vi "Mu_Variance_linearCombinaison.vi"(11 "elements":cluster{"Intensity Graph 3":u8[][]}[][](array[cluster])) -> ()   [LabVIEW 2018, in "statistics.lvlib"]
uses:
  statistics.lvlib
panel:
  in  "Hologram array":dbl[](array[numeric])=[0.0, 0.25, 0.5, 0.75]
  out "subarray":cluster{"Intensity Graph 3":u8[][]}[](array[cluster])
  out "element":i32
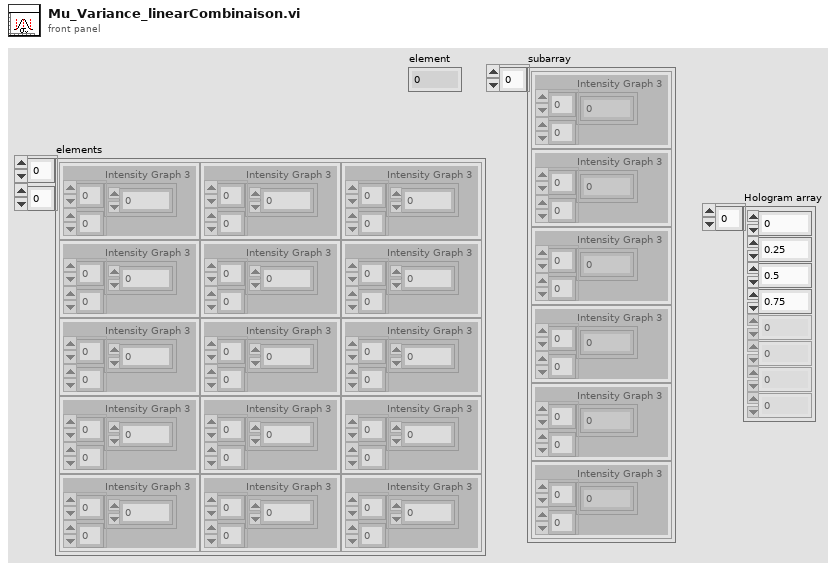
[diagram p1: front panel]
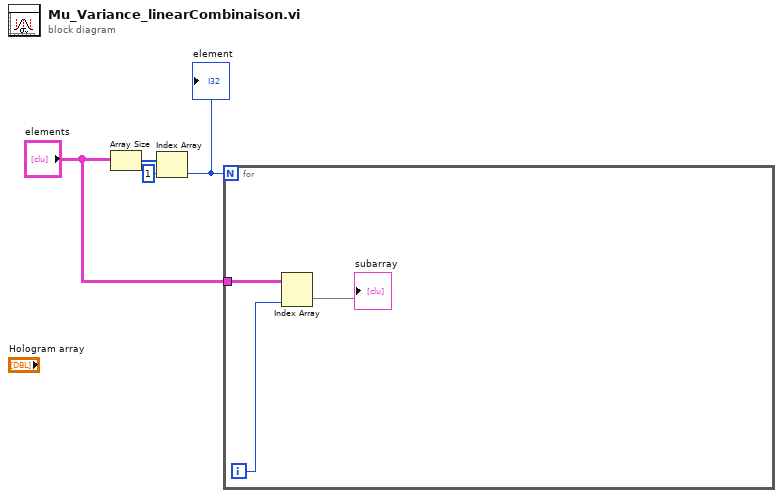
[diagram p0: block diagram]
diagram:
  n1 = Array Size(array="elements") -> (size(s)=w4:i32[])
  n2 = Index Array(array=w4, index=1) -> (element=w2:i32)
  "element" <- w2
  n3 = for {
    N: w2 -> [_]
    tunnel: "elements" -> [w7]
    i -> [w6]
    n4 = Index Array(array=w7, index (col)=w6) -> (element=→"subarray":cluster{"Intensity Graph 3":u8[][]}[])  [unwired: 1 in]
  }
